vi "Debug - TCP - Append New Line to Log.vi"(9 "Transmission Log":string) -> ()   [LabVIEW 2017, in "Communications Library.lvlib"]
doc: "Add a line to the TCP debug log file. The line should include a placeholder, where the IP and port number will later be written.\n\nNote: This VI must be non-reentrant, in order to avoid simulatenous writes to the same file by multiple threads."
uses:
  Communications Library.lvlib
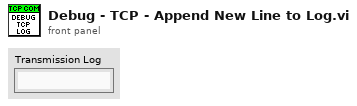
[diagram p1: front panel]
types:
  T1 = enum16{"open", "replace", "create", "open or create", "replace or create", "replace or create with confirmation"}
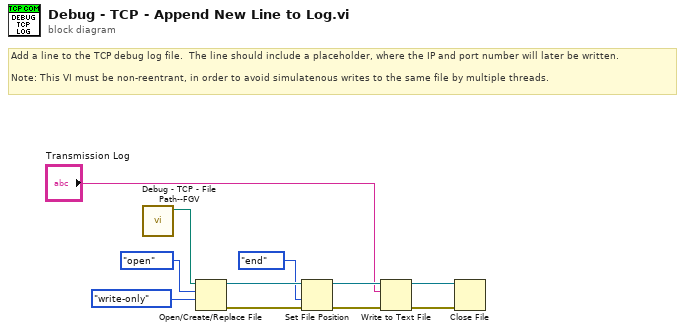
[diagram p0: block diagram]
diagram:
  # "Add a line to the TCP debug log file.  The line should include a placeholder, where the IP and port number will later be written.\n\nNote: This VI must be non-reentrant, in order to avoid simulatenous writes to the same file by multiple threads."
  n1 = call "Debug - TCP - File Path--FGV.vi"() -> ("Debug Pathname"=w1:path)  [unwired: 11 in]
  n2 = Open/Create/Replace File(file path (use dialog)=w1, operation (0:open)=T1."open", access (0:read/write)=enum16{"read/write", "read-only", "write-only"}."write-only") -> (refnum out=w10:refnum<file>, error out=w11:errorcluster)  [unwired: 3 in, 1 out]
  n3 = Set File Position(refnum=w10, from (0:start)=enum16{"start", "end", "current"}."end", error in=w11) -> (refnum out=w5:refnum<file>, error out=w6:errorcluster)  [unwired: 1 in]
  n4 = Write to Text File(file (use dialog)=w5, text="Transmission Log", error in=w6) -> (refnum out=w3:refnum<file>, error out=w4:errorcluster)  [unwired: 1 in, 1 out]
  n5 = Close File(refnum=w3, error in=w4) -> ()  [unwired: 2 out]
